vi "20.vi"() -> ()   [LabVIEW 2021]
panel:
  out "Sum of Digits":u64
  out "N!":u8[](array[numeric])
  in  "N":u64
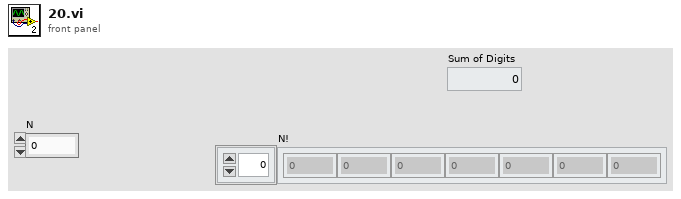
[diagram p1: front panel]
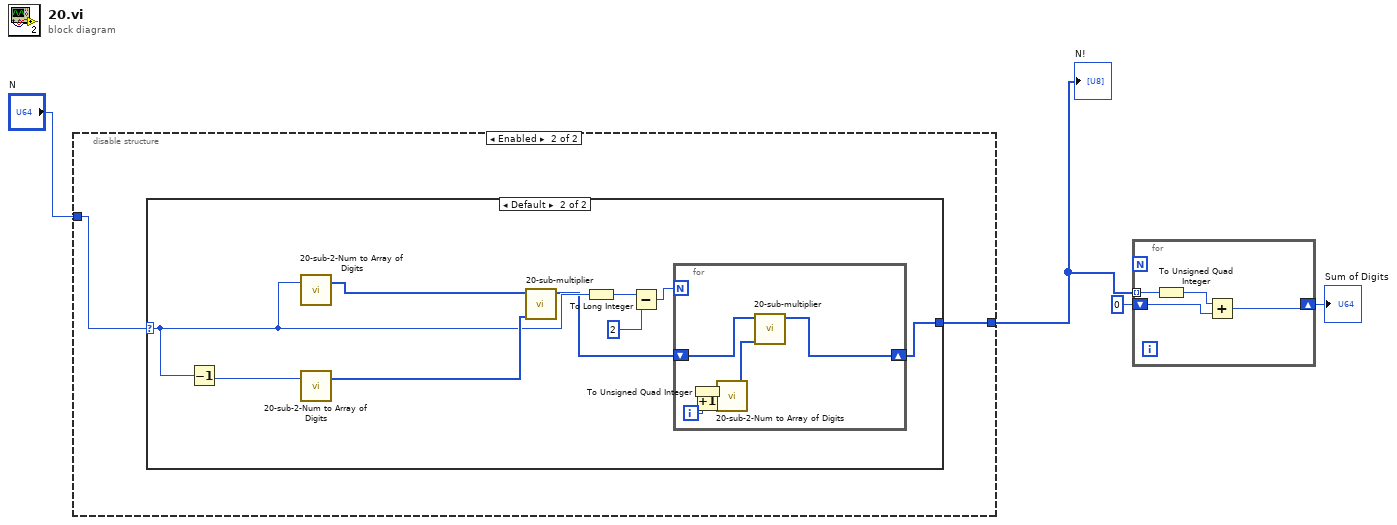
[diagram p0: block diagram]
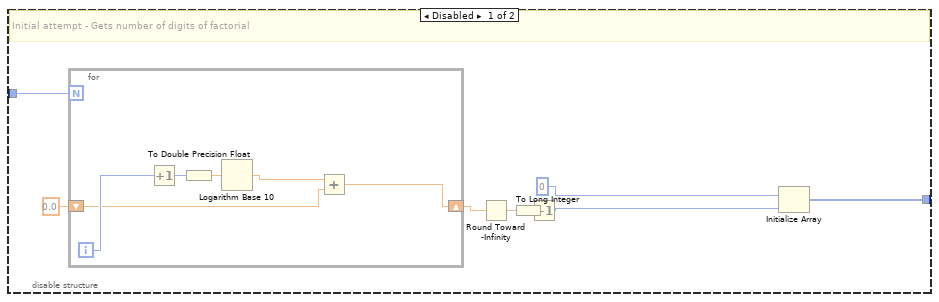
[diagram p2: hidden frame]
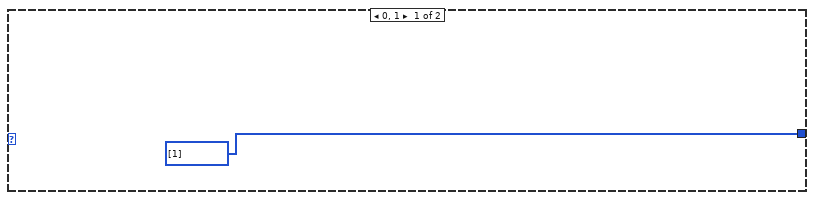
[diagram p3: hidden frame]
diagram:
  n1 = disable-structure shown="Enabled" {
    disable-tunnel: "N" -> [w12 w20]
    disable-tunnel: [w7 w19] -> w3
    frame Disabled {
      # "Initial attempt - Gets number of digits of factorial"
      n2 = for {
        N: w12 -> [_]
        shift-right: [w14] -> w10
        shift-left: 0.0 -> [w15]
        i -> [w18]
        n3 = Increment(x=w18) -> (x+1=w17:i32)
        n4 = To Double Precision Float(number=w17) -> (double precision float=w16:dbl)
        n5 = Logarithm Base 10(1:w16) -> (0:w13:dbl)
        n6 = Add(x=w13, y=w15) -> (x+y=w14:dbl)
      }
      n7 = Round Toward -Infinity(1:w10) -> (0:w5:dbl)
      n8 = To Long Integer(number=w5) -> (32bit integer=w9:i32)
      n9 = Increment(x=w9) -> (x+1=w6:i32)
      n10 = Initialize Array(u8 0, w6) -> (w7:u8[])
    }
    frame Enabled {
      n11 = case shown="Default" w20 {
        selector: w20 -> [_ w26]
        tunnel: [u8[] [1] ("appended array") w22] -> w19
        frame 0, 1 {
        }
        frame Default {
          n12 = Decrement(x=w26) -> (x-1=w30:u64)
          n13 = call "20-sub-2-Num to Array of Digits.vi"("N"=w26) -> ("N as Array"=w29:u8[])  [unwired: 2 in]
          n14 = call "20-sub-2-Num to Array of Digits.vi"("N"=w30) -> ("N as Array"=w28:u8[])  [unwired: 2 in]
          n15 = call "20-sub-multiplier.vi"("N2"=w28, "N1"=w29) -> ("N1*N2"=w23:u8[])  [unwired: 9 in]
          n16 = To Long Integer(number=w26) -> (32bit integer=w24:i32)
          n17 = Subtract(x=w24, y=2) -> (x-y=w27:i32)
          n18 = for {
            N: w27 -> [_]
            shift-right: [w31] -> w22
            shift-left: w23 -> [w36]
            i -> [w35]
            n19 = Increment(x=w35) -> (x+1=w34:i32)
            n20 = To Unsigned Quad Integer(1:w34) -> (0:w33:u64)
            n21 = call "20-sub-2-Num to Array of Digits.vi"("N"=w33) -> ("N as Array"=w32:u8[])  [unwired: 2 in]
            n22 = call "20-sub-multiplier.vi"("N2"=w32, "N1"=w36) -> ("N1*N2"=w31:u8[])  [unwired: 9 in]
          }
        }
      }
    }
  }
  "N!" <- w3
  n23 = for {
    tunnel: w3 -> [w40] mode=indexing
    shift-right: [w38] -> w1
    shift-left: u64 0 -> [w39]
    n24 = To Unsigned Quad Integer(1:w40) -> (0:w37:u64)
    n25 = Add(x=w37, y=w39) -> (x+y=w38:u64)
  }
  "Sum of Digits" <- w1
